vi "Merge Column.vi"(8 "error in (no error)":errorcluster, 10 "Column to merge from":refnum<class "Column.lvclass">, 11 "Column to merge to":refnum<class "Column.lvclass">) -> (0 "error out":errorcluster, 3 "Merged column":refnum<class "Column.lvclass">)   [LabVIEW 2020]
uses:
  Column.lvclass
  C:/Users/User/Desktop/Raman Program/Database OOP/source/Database OOP/Basic Columns/Column Class/Column.lvclass
  C:/Users/User/Desktop/Raman Program/Database OOP/source/Database OOP/Column Interface/Column Interface Class/Column Interface.lvclass
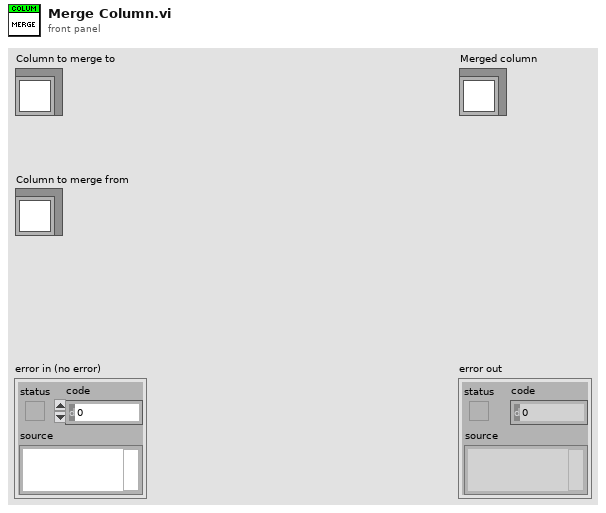
[diagram p1: front panel]
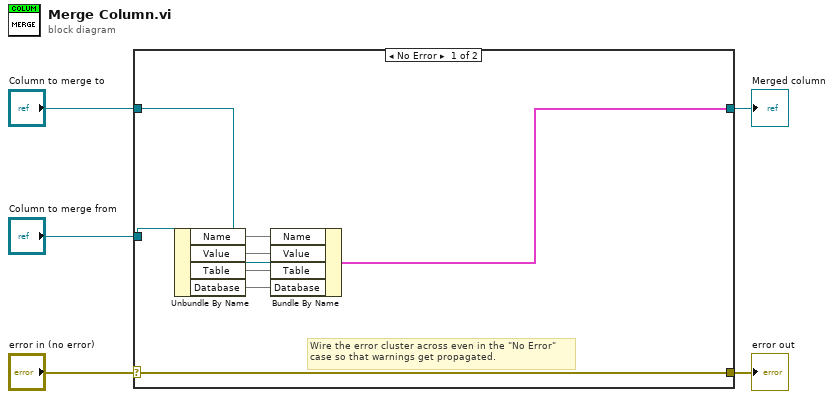
[diagram p0: block diagram]
diagram:
  n1 = case shown="No Error" "error in (no error)" {
    selector: "error in (no error)" -> [w13 w15]
    tunnel: [w13 w15] -> w4
    tunnel: [w10 w14] -> w2
    tunnel: "Column to merge to" -> [w11 w14]
    tunnel: "Column to merge from" -> [w12 _]
    frame No Error {
      # "Wire the error cluster across even in the \"No Error\"\ncase so that warnings get propagated."
      n2 = Unbundle By Name(w12) -> ("Name"=w9, "Value"=w8, "Table"=w7, "Database"=w6)
      n3 = Bundle By Name(cluster=w11, "Name"=w9, "Value"=w8, "Table"=w7, "Database"=w6) -> (w10:cluster{})
    }
    frame Error {
    }
  }
  "error out" <- w4
  "Merged column" <- w2
